vi "Dispense FN - ON - Setpoints - Static (SubVI).vi"(0 "Main Concentration Setpoint (%)":dbl, 5 "Fill Mass (g)":dbl) -> (16 "Static Setpoint (g)":dbl)   [LabVIEW 2011]
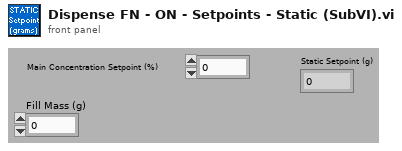
[diagram p1: front panel]
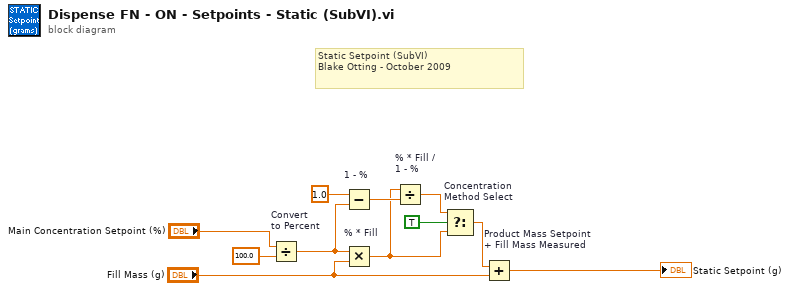
[diagram p0: block diagram]
diagram:
  # "Static Setpoint (SubVI)\nBlake Otting - October 2009"
  n1 = Divide "Convert\nto Percent"(x="Main Concentration Setpoint (%)", y=100.0) -> (x/y=w6:dbl)
  n2 = Subtract "1 - %"(x=1.0, y=w6) -> (x-y=w5:dbl)
  n3 = Multiply "% * Fill"(x=w6, y="Fill Mass (g)") -> (x*y=w1:dbl)
  n4 = Divide "% * Fill /\n1 - %"(x=w1, y=w5) -> (x/y=w3:dbl)
  n5 = Select "Concentration\nMethod Select"(t=w3, s=TRUE, f=w1) -> (s? t:f=w2:dbl)
  n6 = Add "Product Mass Setpoint\n+ Fill Mass Measured"(x=w2, y="Fill Mass (g)") -> (x+y=→"Static Setpoint (g)":dbl)
